vi "Test Discovery Listener.vi"() -> ()   [LabVIEW 2020]
uses:
  Source/epl-network.lvlib
panel:
  out "disconnected":string
  out "connected":T1
  in  "stop":bool
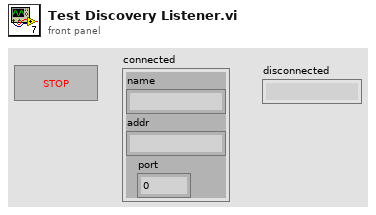
[diagram p1: front panel]
types:
  T1 = cluster{"name":string, "addr":string, "port":u16}
  T2 = typedef "epl-network.lvlib/Discovery Events.ctl" = cluster{"DiscoveredHost":refnum<user-event>, "ExpiredHost":refnum<user-event>}
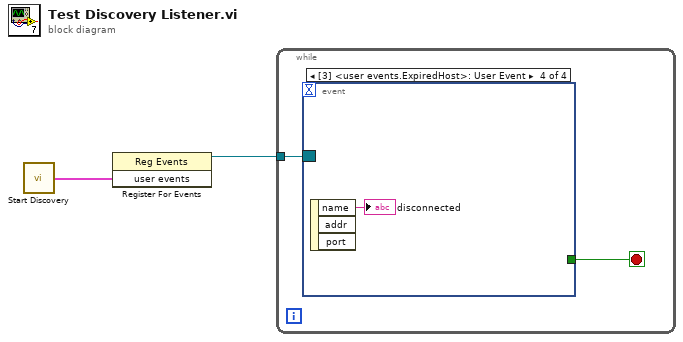
[diagram p0: block diagram]
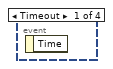
[diagram p2: hidden frame]
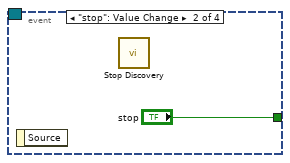
[diagram p3: hidden frame]
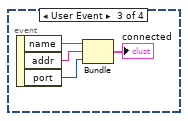
[diagram p4: hidden frame]
diagram:
  n1 = call "Start Discovery.vi"() -> ("user events"=w2:T2)  [unwired: 14 in, 1 out]
  n2 = register-events(w2) -> (reference out=w1:refnum<event-registration>)  [unwired: 2 in, 1 out]
  n3 = while {
    tunnel: w1 -> [w4]
    stop <- w3 stop-if-true
    n4 = event shown="[3] <user events.ExpiredHost>: User Event" {
      selector: w4 -> [_ _ _ _]
      dyn-events: _ -> [_ _ _ _]
      timeout: _ -> [_ _ _ _]
      tunnel: [_ "stop" _ _] -> w3
      event Timeout {
        n5 = event-data() -> ()  [unwired: 1 in, 1 out]
      }
      event "stop": Value Change {
        n6 = event-data() -> ()  [unwired: 1 in, 1 out]
        n7 = call "Stop Discovery.vi"() -> ()  [unwired: 12 in]
      }
      event User Event {
        n8 = event-data() -> ("name"=w9:string, "addr"=w8:string, "port"=w7:u16)  [unwired: 1 in]
        n9 = Bundle("name"=w9, "addr"=w8, "port"=w7) -> (→"connected":T1)  [unwired: 1 in]
      }
      event User Event {
        n10 = event-data() -> ("name"=→"disconnected":string)  [unwired: 1 in, 2 out]
      }
    }
  }
